vi "GetSave.vi"(8 "error in":errorcluster, 10 "ArgIndex(0)":i32, 11 "Args":string[](array[string])) -> (0 "error out":errorcluster, 2 "Arg":string, 3 "Settings.Save":enum16{"off", "on"}(ring))   [LabVIEW 2013]
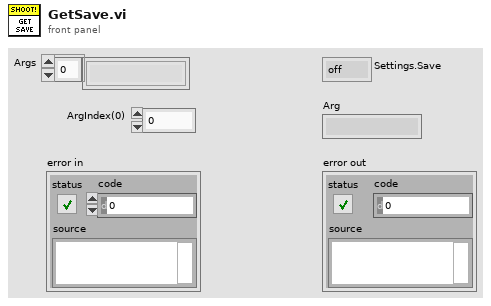
[diagram p1: front panel]
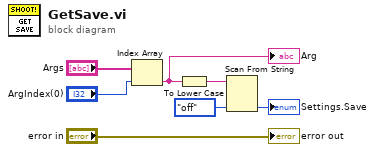
[diagram p0: block diagram]
diagram:
  n1 = Index Array(array="Args", index="ArgIndex(0)") -> (element=w4:string)
  "Arg" <- w4
  n2 = To Lower Case(string=w4) -> (all lower case string=w2:string)
  n3 = Scan From String(input string=w2, default 1=enum16{"off", "on"}."off" ("Settings.Save")) -> (output 1=→"Settings.Save":enum16{"off", "on"})  [unwired: 3 in, 3 out]
  "error out" <- "error in"
